vi "GUI.TabControl.SelectPage.vi"(7 "referenceToControls in":refnum<vi>[](array[refnum]), 8 "error in (no error)":errorcluster, 10 "pageNumber":i32, 11 "tabControlName":string="tabCtl_Pressure") -> (0 "error out":errorcluster, 5 "referenceToControls out":refnum<vi>[](array[refnum]))   [LabVIEW 2019]
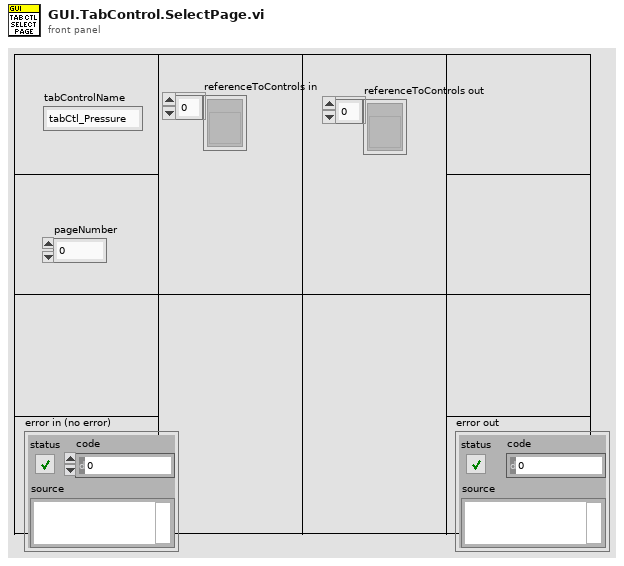
[diagram p1: front panel]
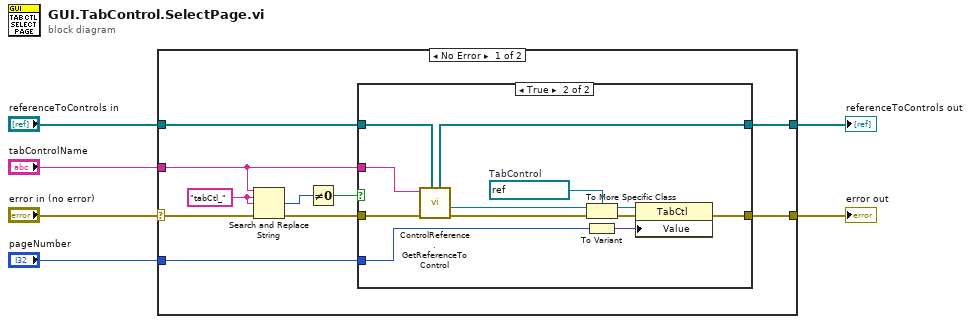
[diagram p0: block diagram]
diagram:
  n1 = case shown="No Error" "error in (no error)" {
    selector: "error in (no error)" -> [w12 w32]
    tunnel: [w16 w32] -> w5
    tunnel: "referenceToControls in" -> [w14 w31]
    tunnel: [w13 w31] -> w3
    tunnel: "pageNumber" -> [w15 _]
    tunnel: "tabControlName" -> [w8 _]
    frame No Error {
      w7 = "tabCtl_"
      n2 = Search and Replace String(input string=w8, search string=w7, replace string=w7, error in=w12) -> (number of replacements=w10:i32, error out=w11:errorcluster)  [unwired: 4 in, 2 out]
      n3 = Not Equal To 0?(x=w10) -> (x != 0?=w9:bool)
      n4 = case shown="True" w9 {
        tunnel: [w17 w29] -> w16
        tunnel: w15 -> [_ w25]
        tunnel: w11 -> [w17 w24]
        tunnel: w14 -> [w18 w20]
        tunnel: [w18 w19] -> w13
        tunnel: w8 -> [_ w23]
        frame False {
        }
        frame True {
          w28 = refnum<vi> refnum  # TabControl
          n5 = call "ControlReference.GetReferenceToControl.vi"("referenceToControls in"=w20, "error in (no error)"=w24, "controlLabelText"=w23) -> ("error out"=w22:errorcluster, "referenceToControl"=w21:refnum<vi>, "referenceToControls out"=w19:refnum<vi>[])  [unwired: 6 in]
          n6 = To More Specific Class(target class=w28, reference=w21, error in=w22) -> (specific class reference=w27:refnum<vi>, error out=w30:errorcluster)
          n7 = To Variant(anything=w25) -> (Variant=w26:variant)
          n8 = property class="TabCtl"(reference=w27, error in=w30, "Value"=w26) -> (error out=w29:errorcluster)  [unwired: 1 out]
        }
      }
    }
    frame Error {
    }
  }
  "error out" <- w5
  "referenceToControls out" <- w3
